vi "Load_from_Project.vi"(8 "error in (no error)":errorcluster, 11 "Object":T1) -> (0 "error out":errorcluster, 3 "Build out":refnum<class "AB_Build.lvclass">)   [LabVIEW 2020, in "AB_Build.lvclass"]
uses:
  <vilib>/AppBuilder/AB_Classes/Build/AB_Build.lvclass
  <resource>/Framework/Providers/API/ItemRef.ctl
  <vilib>/AppBuilder/AB_Classes/Build/AB_Build.lvclass/AB_Build.ctl
  <vilib>/AppBuilder/AB_Classes/Source/AB_Source.lvclass
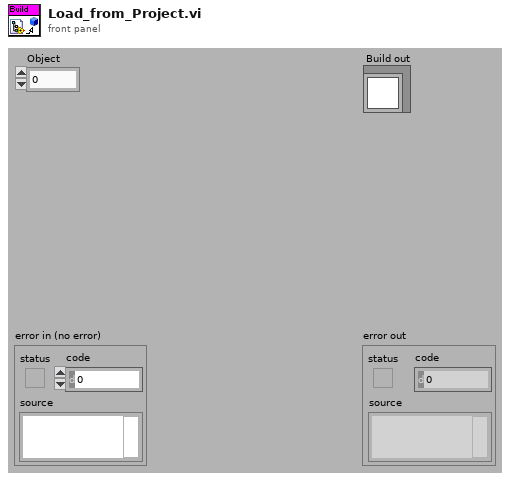
[diagram p1: front panel]
types:
  T1 = typedef "ItemRef.ctl" = u64
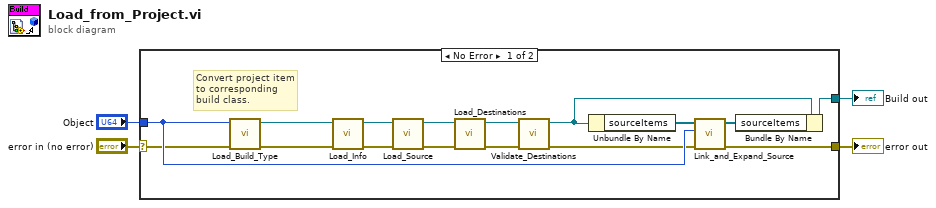
[diagram p0: block diagram]
diagram:
  n1 = case shown="No Error" "error in (no error)" {
    selector: "error in (no error)" -> [w9 w21]
    tunnel: [w19 w21] -> w3
    tunnel: [w18 _] -> w2
    tunnel: "Object" -> [w10 _]
    frame No Error {
      # "Convert project item to corresponding build class."
      n2 = call <vilib>:"Load_Build_Type.vi"("error in (no error)"=w9, "buildObject"=w10) -> ("error out"=w16:errorcluster, "AB_Build out"=w15:refnum<class "AB_Build.lvclass">)  [unwired: 8 in]
      n3 = call-dynamic "Load_Info.vi"("error in (no error)"=w16, "AB_Build in"=w15) -> ("error out"=w11:errorcluster, "AB_Build out"=w12:refnum<class "AB_Build.lvclass">)  [unwired: 8 in]
      n4 = call-dynamic "Load_Source.vi"("error in (no error)"=w11, "AB_Build in"=w12) -> ("error out"=w13:errorcluster, "AB_Build out"=w14:refnum<class "AB_Build.lvclass">)  [unwired: 8 in]
      n5 = call-dynamic "Load_Destinations.vi"("error in (no error)"=w13, "AB_Build in"=w14) -> ("error out"=w6:errorcluster, "AB_Build out"=w8:refnum<class "AB_Build.lvclass">)  [unwired: 8 in]
      n6 = call-dynamic "Validate_Destinations.vi"("error in (no error)"=w6, "AB_Build in"=w8) -> ("error out"=w5:errorcluster, "AB_Build out"=w7:refnum<class "AB_Build.lvclass">)  [unwired: 8 in]
      n7 = Unbundle By Name(w7) -> ("sourceItems"=w20:refnum<class "AB_Source.lvclass">[])
      n8 = call <vilib>:"Link_and_Expand_Source.vi"("error in (no error)"=w5, "Object"=w10, "AB_Source in"=w20) -> ("error out"=w19:errorcluster, "AB_Source out"=w17:refnum<class "AB_Source.lvclass">[])  [unwired: 7 in]
      n9 = Bundle By Name(cluster=w7, "sourceItems"=w17) -> (w18:refnum<class "AB_Build.lvclass">)
    }
    frame Error {
    }
  }
  "error out" <- w3
  "Build out" <- w2
